vi "Presaved Raman curve fitting polybaseline residue.vi"(1 "index":i32, 2 "Initial Guess Coefficient":dbl[](array[numeric])=[1.0, 1.0, 1.0, 1.0, 1.0, 1.0] format="%0.2f", 3 "endX":dbl, 4 "startX":dbl, 5 "Selected data set per point":sgl[][](array[numeric])=[[870.0, 267.0, 0.0], [871.0, 275.5, 0.0], [872.0, 286.5, 0.0], [873.0, 301.5, 0.0], [874.0, 319.5, 0.0], [875.0, 314.0, 0.0], [876.0, 339.5, 0.0], [877.0, 356.5, 0.0], [878.0, 388.5, 0.0], [879.0, 417.5, 0.0], [880.0, 442.0, 0.0], [881.0, 476.5, 0.0], [882.0, 494.5, 0.0], [883.0, 495.5, 0.0], [884.0, 534.0, 0.0], [885.0, 525.5, 0.0], [886.0, 532.0, 0.0], [887.0, 540.0, 0.0], [888.0, 524.0, 0.0], [889.0, 502.5, 0.0], [890.0, 488.5, 0.0], [891.0, 463.5, 0.0], [892.0, 432.0, 0.0], [893.0, 406.0, 0.0], [894.0, 393.0, 0.0], [895.0, 382.0, 0.0], [896.0, 361.0, 0.0], [897.0, 342.0, 0.0], [898.0, 328.5, 0.0], [899.0, 318.0, 0.0]] format="%#_8g") -> (0 "Coefficients":dbl[](array[numeric])=[455.50070847704825, 2012.484427388756, -6.643317132800543, 872.0401845675163] format="%0.2f")   [LabVIEW 2015]
doc: "Demonstrates how the Levenberg-Marquardt algorithm can determine the least squares set of coefficients that best fit the set of input data points(X,Y) as expressed by a nonlinear function y=f(x,a) where a is the set of coefficients.\n\nNote: You must have the LabVIEW Full or Professional Development Systems to run this example."
uses:
  <vilib>/gmath/NumericalOptimization/Nonlinear Curve Fit LM.vi
  <vilib>/gmath/NI_Gmath.lvlib
panel:
  out "residue":dbl=2012.484427388756
  out "a4":dbl=2012.484427388756
  out "a3":dbl=2012.484427388756
  out "a2":dbl=2012.484427388756
  out "error out":errorcluster
  out "a1":dbl=2012.484427388756
  out "?":T1(graph)
  # "Multi-linear regression Algorithm"
  # "Data and Fitting results plot"
  # "Fitting Results"
  # "Version 1.0\nAVM"
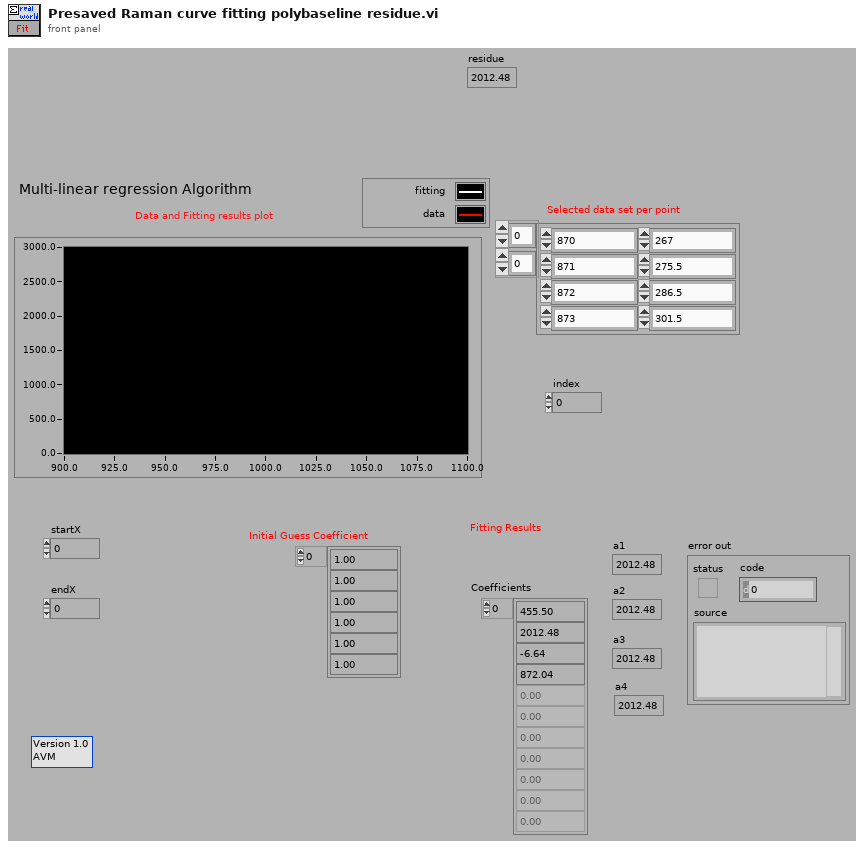
[diagram p1: front panel]
types:
  T1 = cluster{"Selected data set per point":sgl[], "best nonlinear fit":dbl[]}[]
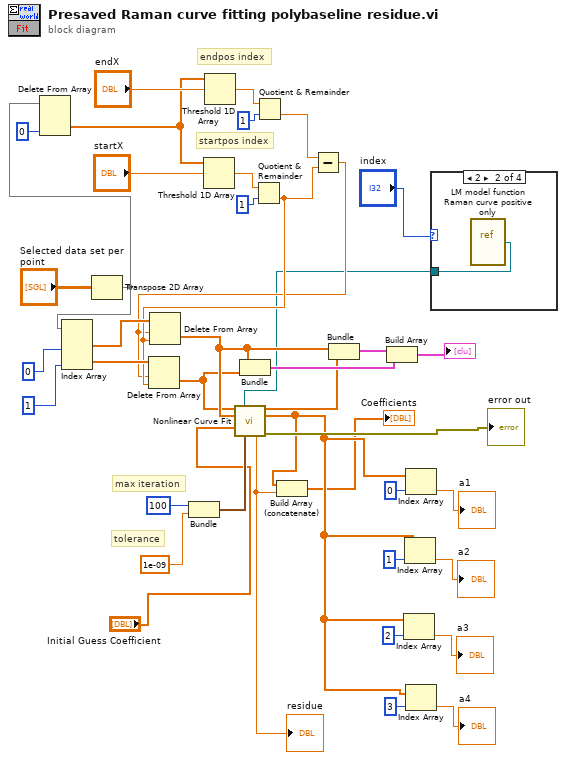
[diagram p0: block diagram]
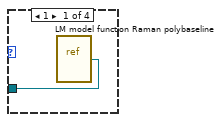
[diagram p2: hidden frame]
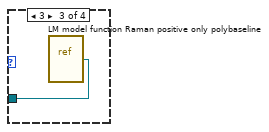
[diagram p3: hidden frame]
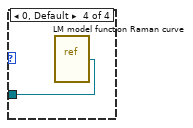
[diagram p4: hidden frame]
diagram:
  # "endpos index"
  # "startpos index"
  # "tolerance"
  # "max iteration"
  n1 = Transpose 2D Array(2D array="Selected data set per point") -> (transposed array=w18:sgl[][])
  n2 = Delete From Array(array=w18, index (col)=0 ("disabled index (col)")) -> (deleted portion=w20:sgl[])  [unwired: 2 in, 1 out]
  n3 = Index Array(array=w18, index (col) #1=0 ("disabled index (col)"), index (col) #2=1 ("index (col)")) -> (element #1=w14:sgl[], element #2=w13:sgl[])  [unwired: 2 in]
  n4 = Bundle("index (col)"=100, "index (col)"=1e-09) -> (w34:cluster{"index (col)":i32, "index (col)":dbl})  [unwired: 1 in]
  n5 = Threshold 1D Array(2:"startX", 3:w20) -> (0:w27:sgl)  [unwired: 1 in]
  n6 = Threshold 1D Array(2:"endX", 3:w20) -> (0:w24:sgl)  [unwired: 1 in]
  n7 = Quotient & Remainder(x=w27, y=1) -> (floor(x/y)=w12:sgl)  [unwired: 1 out]
  n8 = Quotient & Remainder(x=w24, y=1) -> (floor(x/y)=w19:sgl)  [unwired: 1 out]
  n9 = Subtract(x=w19, y=w12) -> (x-y=w11:sgl)
  n10 = Delete From Array(array=w13, length=w11, index=w12) -> (deleted portion=w10:sgl[])  [unwired: 1 out]
  n11 = Delete From Array(array=w14, length=w11, index=w12) -> (deleted portion=w15:sgl[])  [unwired: 1 out]
  n12 = Bundle(w15, w10) -> (w40:cluster{sgl[], sgl[]})  [unwired: 1 in]
  n13 = case shown="2" "index" {
    tunnel: [w42 w43 w44 w45] -> w7
    frame 1 {
      n14 = vi-ref "LM model function Raman polybaseline.vi"() -> (w42:refnum<vi>)
    }
    frame 2 {
      n15 = vi-ref "LM model function Raman curve positive only.vi"() -> (w43:refnum<vi>)
    }
    frame 3 {
      n16 = vi-ref "LM model function Raman positive only polybaseline.vi"() -> (w44:refnum<vi>)
    }
    frame 0, Default {
      n17 = vi-ref "LM model function Raman curve.vi"() -> (w45:refnum<vi>)
    }
  }
  n18 = call-poly <vilib>:"Nonlinear Curve Fit.vi"("Y"=w10, "f(x,a)"=w7, "X"=w15, "initial parameters"="Initial Guess Coefficient", "termination"=w34) -> ("best nonlinear fit"=w33:dbl[], "best fit parameters"=w3:dbl[], "residue"=w2:dbl, "error out"=→"error out":errorcluster)  [unwired: 5 in, 2 out]
  "residue" <- w2
  n19 = Build Array (concatenate)(w3, w2) -> (→"Coefficients":dbl[])
  n20 = Bundle(w15, "best nonlinear fit"=w33) -> (w41:cluster{sgl[], "best nonlinear fit":dbl[]})  [unwired: 1 in]
  n21 = Build Array(w41, w40) -> (→"?":cluster{sgl[], "best nonlinear fit":dbl[]}[])
  n22 = Index Array(array=w3, index=2) -> (element=→"a3":dbl)
  n23 = Index Array(array=w3, index=1) -> (element=→"a2":dbl)
  n24 = Index Array(array=w3, index=0) -> (element=→"a1":dbl)
  n25 = Index Array(array=w3, index=3) -> (element=→"a4":dbl)
